vi "Symmetric Window (CDB).vi"(9 "window parameter":dbl=nan, 10 "window":T1 items=["Rectangle"=0, "Hanning"=1, "Hamming"=2, "Blackman-Harris"=3, "Exact Blackman"=4, "Blackman"=5, "Flat Top"=6, "4 Term B-Harris "=7, "7 Term B-Harris"=8, "Low Sidelobe"=9, "Blackman Nuttall"=11, "Triangle"=30, "Bartlett-Hanning"=31, "Bohman"=32, "Parzen"=33, "Welch"=34, "Kaiser"=60, "Dolph-Chebyshev"=61, "Gaussian"=62], 11 "X":cdb[](array[numeric])) -> (0 "error":i32, 3 "Windowed X":cdb[](array[numeric]))   [LabVIEW 2017, in "NI_AALPro.lvlib"]
doc: "Applies a symmetric window to the input sequence <B>X</B>. Wire data to the <B>X</B> input to determine the polymorphic instance to use or manually select the instance."
uses:
  NI_AALPro.lvlib
  windowTd.ctl
  lvanlys.dll
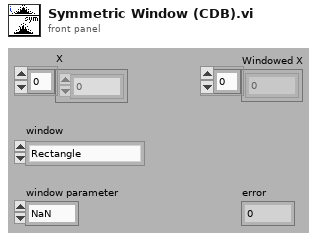
[diagram p1: front panel]
types:
  T1 = typedef "NI_AALPro.lvlib/windowTd.ctl" = u32
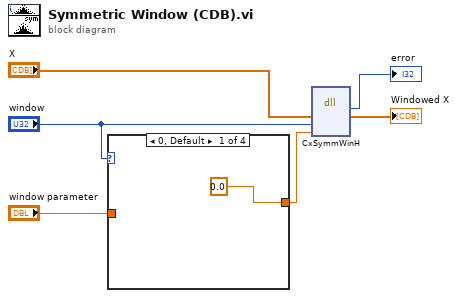
[diagram p0: block diagram]
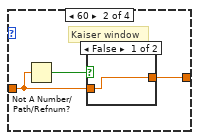
[diagram p2: hidden frame]
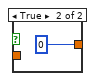
[diagram p3: hidden frame]
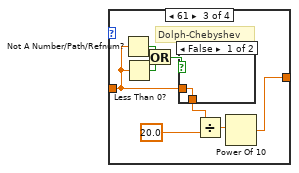
[diagram p4: hidden frame]
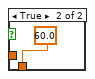
[diagram p5: hidden frame]
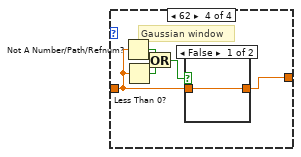
[diagram p6: hidden frame]
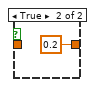
[diagram p7: hidden frame]
diagram:
  n1 = case shown="0, Default" "window" {
    tunnel: [0.0 ("s(db)") w10 w18 w27] -> w3
    tunnel: "window parameter" -> [_ w9 w16 w25]
    frame 0, Default {
    }
    frame 60 {
      # "Kaiser window"
      n2 = Not A Number/Path/Refnum?(number/path/refnum=w9) -> (NaN/Path/Refnum?=w8:bool)
      n3 = case shown="False" w8 {
        tunnel: [w11 0] -> w10
        tunnel: w9 -> [w11 _]
        frame False {
        }
        frame True {
        }
      }
    }
    frame 61 {
      # "Dolph-Chebyshev"
      n4 = Not A Number/Path/Refnum?(number/path/refnum=w16) -> (NaN/Path/Refnum?=w15:bool)
      n5 = Less Than 0?(x=w16) -> (x < 0?=w14:bool)
      n6 = Or(x=w15, y=w14) -> (x .or. y?=w13:bool)
      n7 = case shown="False" w13 {
        tunnel: [w21 60.0 ("y")] -> w17
        tunnel: w16 -> [w21 _]
        frame False {
        }
        frame True {
        }
      }
      n8 = Divide(x=w17, y=20.0) -> (x/y=w19:dbl)
      n9 = Power Of 10(x=w19) -> (10^x=w18:dbl)
    }
    frame 62 {
      # "Gaussian window"
      n10 = Not A Number/Path/Refnum?(number/path/refnum=w25) -> (NaN/Path/Refnum?=w26:bool)
      n11 = Less Than 0?(x=w25) -> (x < 0?=w24:bool)
      n12 = Or(x=w26, y=w24) -> (x .or. y?=w23:bool)
      n13 = case shown="False" w23 {
        tunnel: w25 -> [w28 _]
        tunnel: [w28 0.2 ("para")] -> w27
        frame False {
        }
        frame True {
        }
      }
    }
  }
  n14 = dll-call lib="C:/Program Files/National Instruments/LabVIEW 2017/resource/lvanlys.*" fn="CxSymmWinH"("X"="X", "winType"="window", "para"=w3) -> (→"error":i32, "X"=→"Windowed X":cdb[])  [unwired: 5 in, 2 out]
